vi "MAC-Tester.vi"() -> ()   [LabVIEW 2017]
uses:
  FPGANic/Source.Machine.Settings.ctl
  MAC.Events.ctl
  <vilib>/FPGAPlugInAG/PXIe-6592R/niLvFpga_Open_PXIe-6592R.vi
  <vilib>/rvi/interface/common/dynamic/niFpgaDynamicAddResources.vi
  Globals.vi
  <vilib>/Utility/error.llb/Error Cluster From Error Code.vi
  <vilib>/rvi/errors/niLvFpgaAdjustHostInterfaceError.vi
  <vilib>/FPGAPlugInAG/Dynamic/niLvFpga_Close_Dynamic.vi
  <vilib>/rvi/interface/nirviOpenFPGA/nirviOpenFPGA.xnode
  FPGA Bitfiles/Fpga-Mac-Top.lvbitx
  <vilib>/rvi/interface/nirviMethod/nirviMethod.xnode
  <vilib>/rvi/interface/nirviCloseFPGA/nirviCloseFPGA.xnode
  <vilib>/rvi/errors/niLvFpgaMergeErrorWithErrorCode.vi
  <vilib>/FPGAPlugInAG/Dynamic/niLvFpga_ReadFifo_Dynamic.vi
  <vilib>/FPGAPlugInAG/Dynamic/niLvFpga_WriteFifo_Dynamic.vi
panel:
  in  "MAC & IP":T1={"MAC Address"=[0, 1, 2, 3, 4, 5], "IP Address"=[10, 0, 1, 101]} {"MAC Address" format="%.0x"}
  in  "Ethernet II Params":T2={"Destination MAC"=[0, 2, 201, 85, 8, 68], "Source MAC"=[0, 1, 2, 3, 4, 5], "EtherType"=2048} {"Destination MAC" format="%.0x"; "Source MAC" format="%.02x"; "EtherType" format="%.0x"}
  in  "IPv4 Params":T3={"Destination IP"=[10, 0, 1, 100], "Source IP"=[10, 0, 1, 101], "Protocol"=17}
  in  "UDP Params":T4={"Source Port"=35312, "Destination Port"=35312, "Payload"="ABCD"}
  out "Status":string
  out "error out":errorcluster
  in  "Exit":bool
  in  "Transmit Packet":bool
  in  "Read Packet":bool
  out "RX Data":u8[](array[numeric])=[0, 1, 2, 3, 4, 5, 0, 2, 201, 85, 8, 68, 8, 6, 0, 1, 8, 0, 6, 4, 0, 1, 0, 2, 201, 85, 8, 68, 10, 0, 1, 100, 0, 0, 0, 0, 0, 0, 10, 0, 1, 101, 0, 0, 0, 0, 0, 0, 0, 0, 0, 0, 0, 0, 0, 0, 0, 0, 0, 0, 28, 161, 25, 173] format="%.0x"
  in  "error in":errorcluster
  # "Send Parameters"
  # "Received Data"
  # "NIC Parameters"
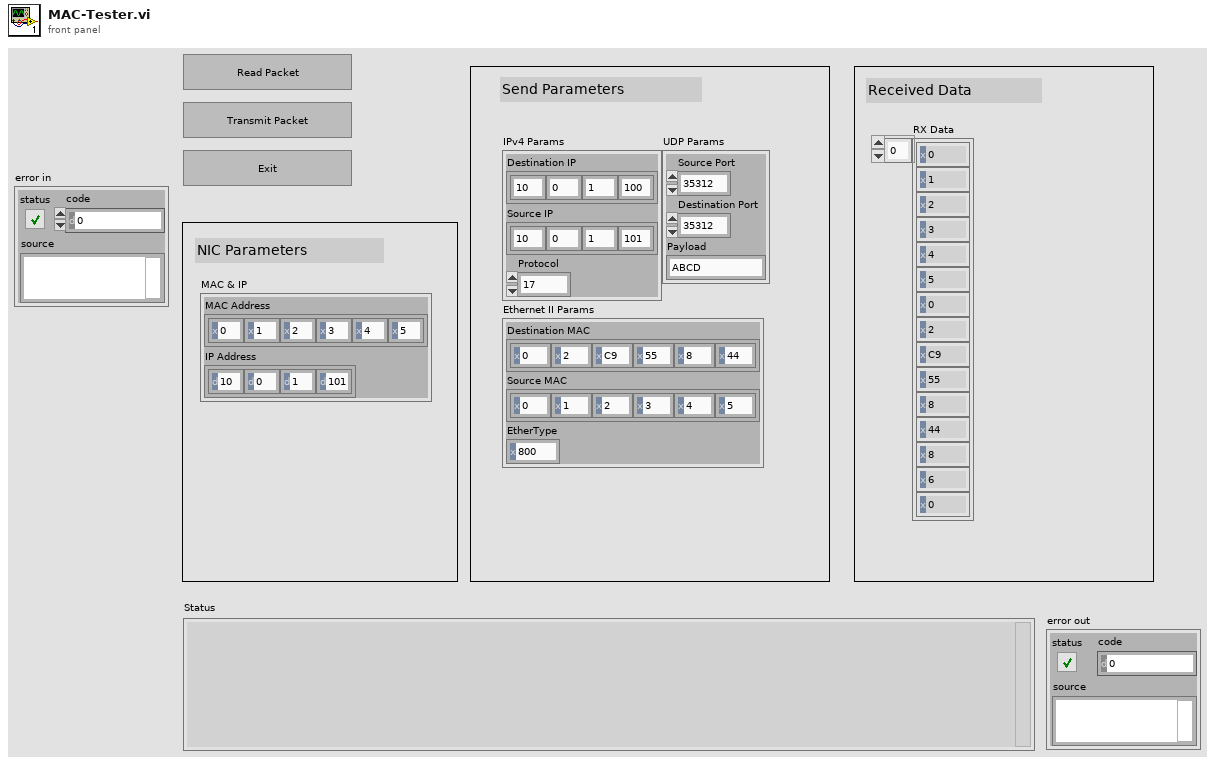
[diagram p1: front panel]
types:
  T1 = typedef "Source.Machine.Settings.ctl" = cluster{"MAC Address":u8[], "IP Address":u8[]}
  T2 = cluster{"Destination MAC":u8[], "Source MAC":u8[], "EtherType":u16}
  T3 = cluster{"Destination IP":u8[], "Source IP":u8[], "Protocol":u8}
  T4 = cluster{"Source Port":u16, "Destination Port":u16, "Payload":string}
  T5 = typedef "MAC.Events.ctl" = enum16{"Open FPGA", "Close FPGA", "Poll RX", "Transmit Packet"}
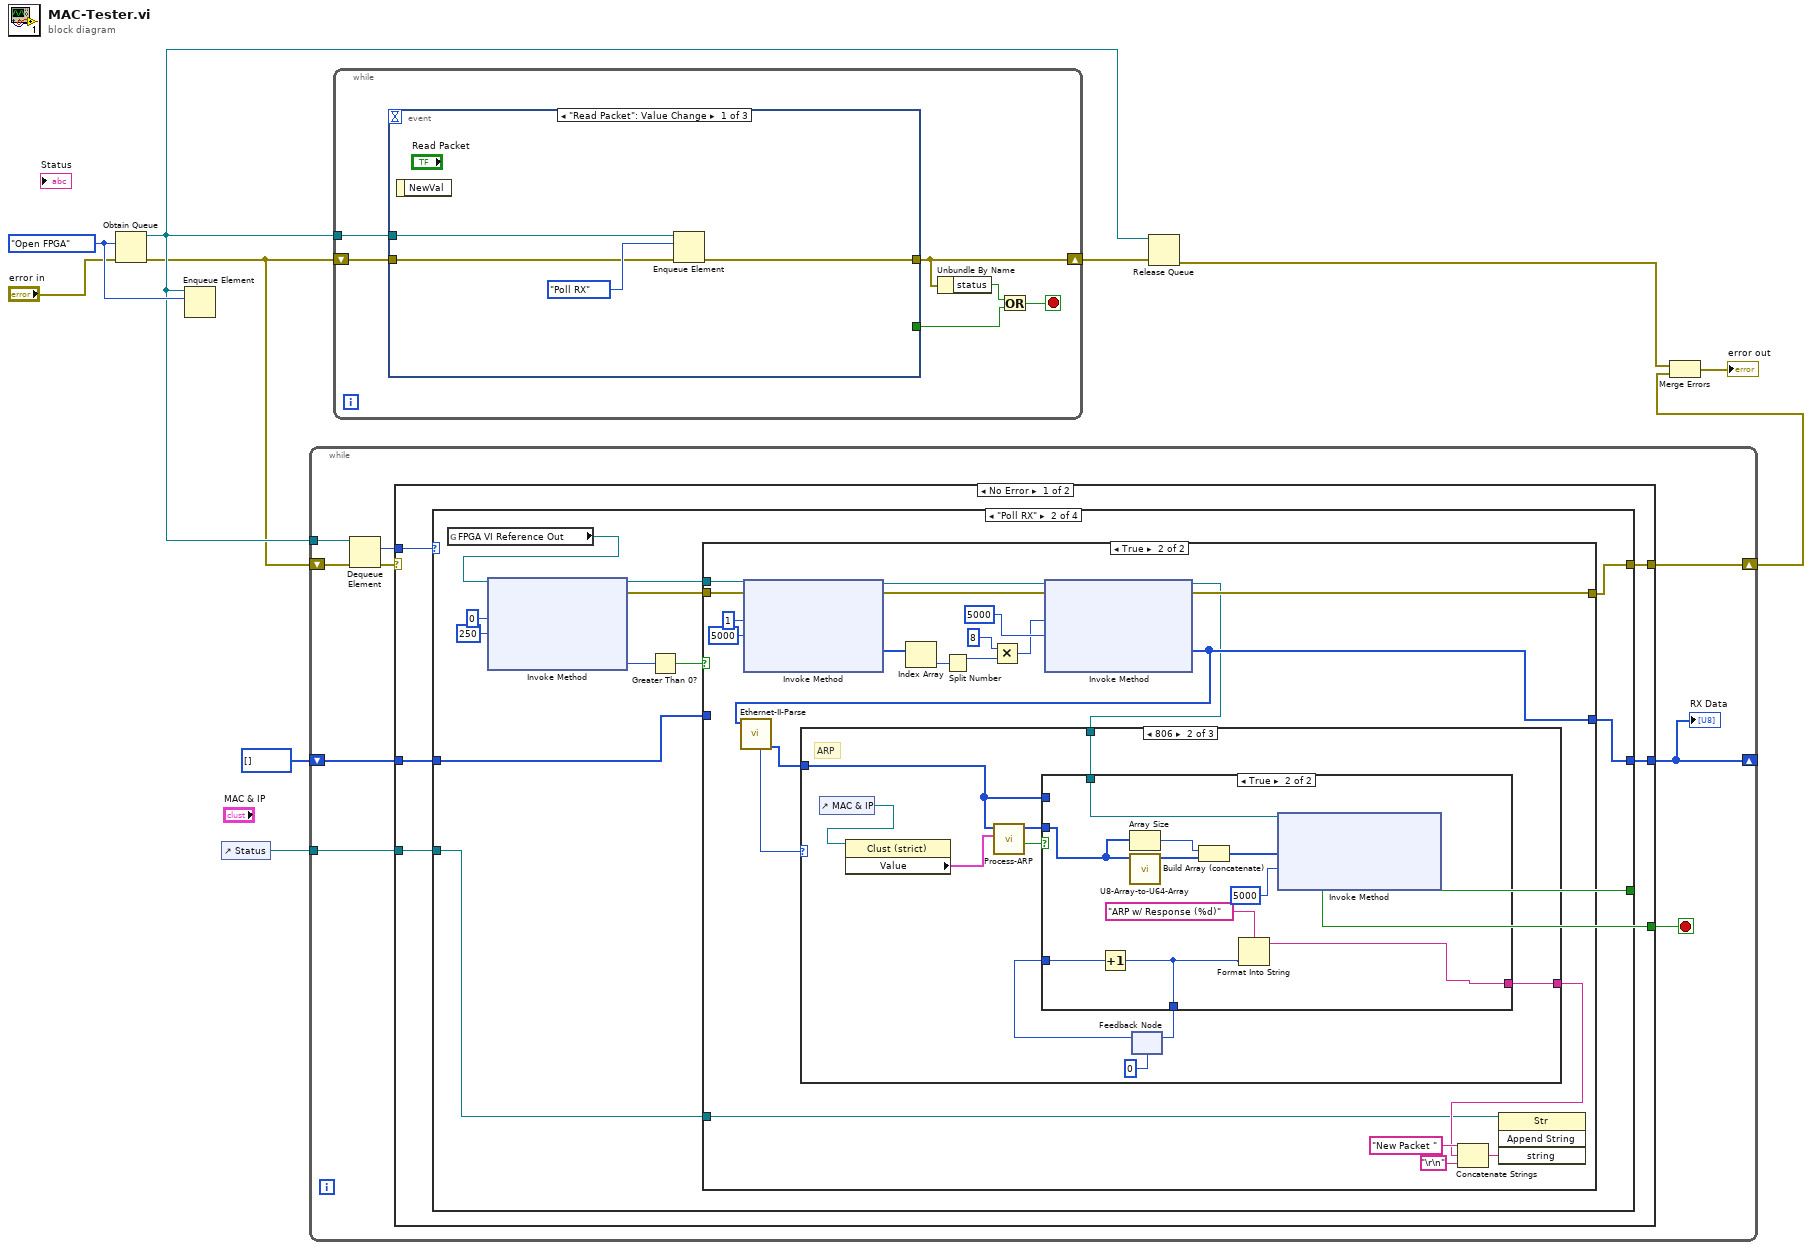
[diagram p0: block diagram]
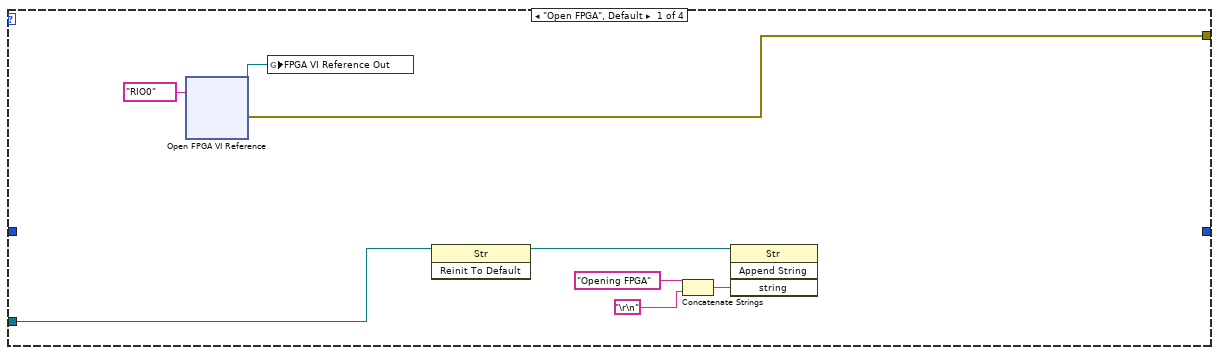
[diagram p2: hidden frame]
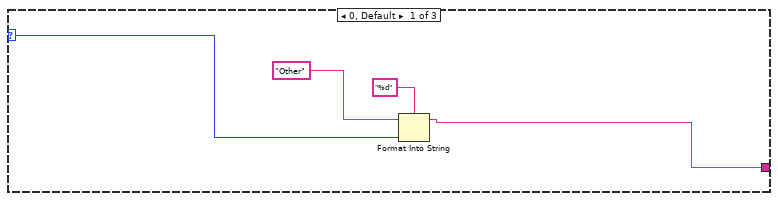
[diagram p4: hidden frame]
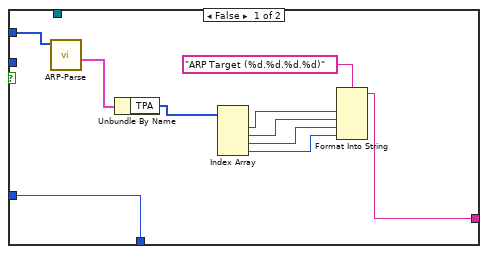
[diagram p5: hidden frame]
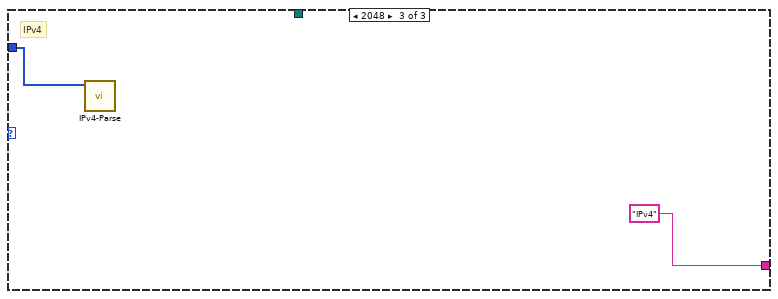
[diagram p6: hidden frame]
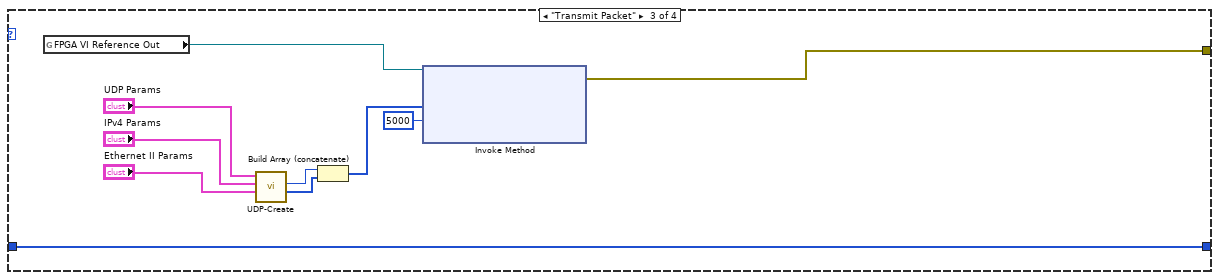
[diagram p7: hidden frame]
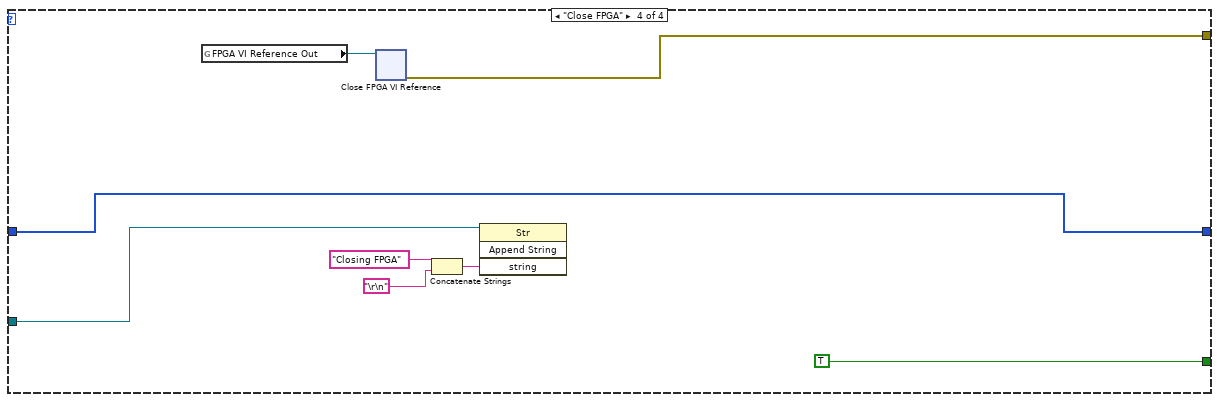
[diagram p8: hidden frame]
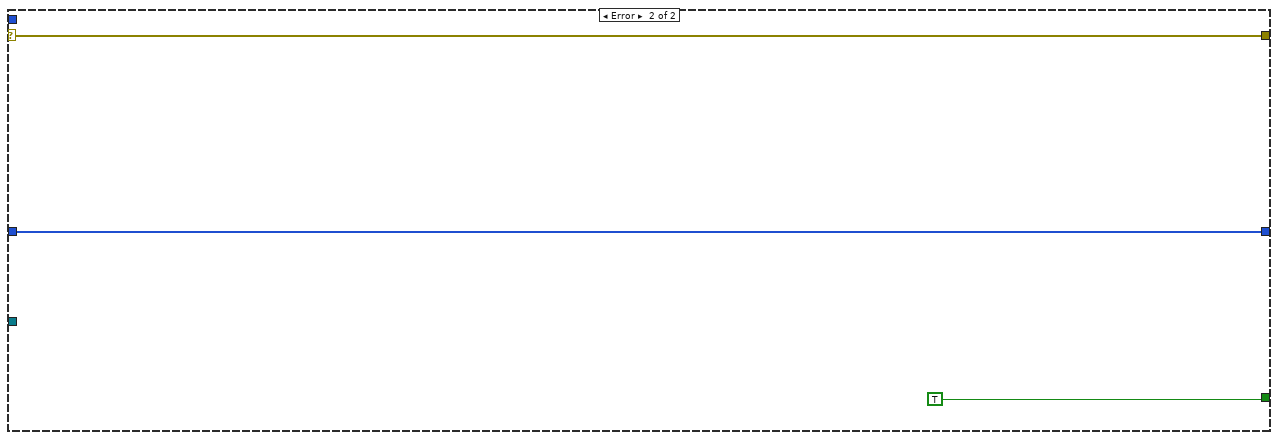
[diagram p9: hidden frame]
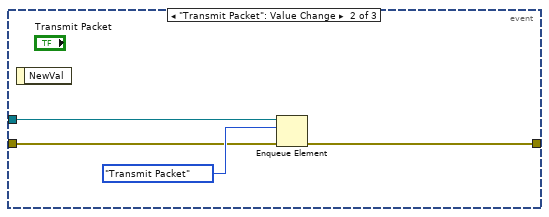
[diagram p10: hidden frame]
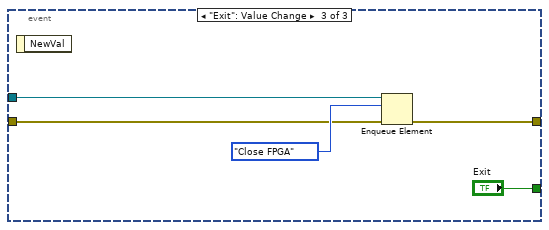
[diagram p11: hidden frame]
diagram:
  w10 = MAC.Events."Open FPGA"
  n1 = Obtain Queue(element data type=w10, error in (no error)="error in") -> (queue out=w8:refnum<queue>, error out=w6:errorcluster)  [unwired: 3 in, 1 out]
  n2 = Enqueue Element(queue=w8, element=w10) -> ()  [unwired: 2 in, 3 out]
  n3 = control-ref of="Status"() -> (w4:refnum<vi>)
  n4 = while {
    tunnel: w8 -> [w19]
    shift-right: [w13] -> w3
    shift-left: w6 -> [w15]
    shift-right: [w12] -> _
    shift-left: u8[] [] -> [w14]
    tunnel: w4 -> [w11]
    stop <- w16 stop-if-true
    n5 = Dequeue Element(queue=w19, error in (no error)=w15) -> (element=w17:T5, error out=w18:errorcluster)  [unwired: 1 in, 2 out]
    n6 = case shown="No Error" w18 {
      selector: w18 -> [_ w123]
      tunnel: w17 -> [w25 _]
      tunnel: [w24 TRUE] -> w16
      tunnel: [w23 w123] -> w13
      tunnel: w14 -> [w22 w124]
      tunnel: [w21 w124] -> w12
      tunnel: w11 -> [w20 _]
      frame No Error {
        n7 = case shown="\"Poll RX\"" w25 {
          tunnel: [_ _ _ TRUE] -> w24
          tunnel: [w33 w36 w106 w121] -> w23
          tunnel: w22 -> [_ w38 w114 w116]
          tunnel: [_ w37 w114 w116] -> w21
          tunnel: w20 -> [w29 w35 _ w117]
          frame "Open FPGA", Default {
            n8 = xnode "Open FPGA VI Reference"("resource name"=tag "RIO0") -> ("FPGA VI Reference Out"=w26:refnum<k20>, "error out"=w33:errorcluster)  [unwired: 1 in]
            n9 = global write "Globals.vi" "FPGA VI Reference Out"(w26) -> ()
            n10 = invoke class="Str" method="Reinit To Default"(reference=w29) -> (reference out=w28:refnum<vi>)  [unwired: 2 in, 2 out]
            n11 = Concatenate Strings("Opening FPGA" ("string"), "\r\n") -> (w32:string)
            n12 = invoke class="Str" method="Append String"(reference=w28, "string"=w32) -> ()  [unwired: 2 in, 4 out]
          }
          frame "Poll RX" {
            n13 = global read "Globals.vi" "FPGA VI Reference Out"() -> (w34:refnum<k20>)
            n14 = xnode "Invoke Method"("FPGA VI Reference In"=w34, "Number of Elements"=u32 0, "Timeout (ms)"=250) -> ("FPGA VI Reference Out"=w40:refnum<k20>, "error out"=w39:errorcluster, "Elements Remaining"=w42:u32)  [unwired: 1 in, 1 out]
            n15 = Greater Than 0?(x=w42) -> (x > 0?=w41:bool)
            n16 = case shown="True" w41 {
              tunnel: w40 -> [_ w66]
              tunnel: w39 -> [w45 w65]
              tunnel: w38 -> [w46 _]
              tunnel: [w46 w50] -> w37
              tunnel: [w45 w59] -> w36
              tunnel: w35 -> [_ w48]
              frame False {
              }
              frame True {
                n17 = xnode "Invoke Method"("FPGA VI Reference In"=w66, "error in"=w65, "Number of Elements"=u32 1, "Timeout (ms)"=5000) -> ("FPGA VI Reference Out"=w62:refnum<k20>, "error out"=w63:errorcluster, "Data"=w64:u32[])  [unwired: 1 out]
                n18 = Index Array(array=w64) -> (element=w61:u32)  [unwired: 1 in]
                n19 = Split Number(x=w61) -> (hi(x)=w55:u16)  [unwired: 1 out]
                n20 = Multiply(x=u16 8 ("y"), y=w55) -> (x*y=w58:u16)
                n21 = xnode "Invoke Method"("FPGA VI Reference In"=w62, "error in"=w63, "Number of Elements"=w58, "Timeout (ms)"=5000) -> ("FPGA VI Reference Out"=w49:refnum<k20>, "error out"=w59:errorcluster, "Data"=w50:u8[])  [unwired: 1 out]
                n22 = call "Ethernet-II-Parse.vi"("Input Frame"=w50) -> ("Payload"=w47:u8[], "EtherType"=w53:u16)  [unwired: 6 in, 3 out]
                n23 = case shown="806" w53 {
                  selector: w53 -> [w72 _ _]
                  tunnel: [w69 w82 "IPv4" ("string")] -> w51
                  tunnel: w47 -> [_ w75 w103]
                  tunnel: w49 -> [_ w79 _]
                  frame 0, Default {
                    n24 = Format Into String(format string="%d", initial string="Other" ("string"), w72) -> (resulting string=w69:string)  [unwired: 1 in, 1 out]
                  }
                  frame 2054 {
                    # "ARP"
                    n25 = control-ref of="MAC & IP"() -> (w73:refnum<vi>)
                    n26 = property class="Clust (strict)"(reference=w73) -> ("Value"=w74:T1)  [unwired: 1 in, 2 out]
                    n27 = call "Process-ARP.vi"("Source Machine\nSettings"=w74, "Frame (in)"=w75) -> ("Response\nNeeded?"=w81:bool, "ARP Response"=w80:u8[])  [unwired: 8 in]
                    n28 = feedback #1(0) -> (w76:i32)
                    n29 = case shown="True" w81 {
                      tunnel: [w89 w93] -> w82
                      tunnel: w80 -> [_ w100]
                      tunnel: w79 -> [_ w101]
                      tunnel: [w92 w95] -> w77
                      tunnel: w76 -> [w92 w96]
                      tunnel: w75 -> [w91 _]
                      frame False {
                        n30 = call "ARP-Parse.vi"("Frame (in)"=w91) -> ("Target"=w88:cluster{"THA":u8[], "TPA":u8[]})  [unwired: 8 in, 2 out]
                        n31 = Unbundle By Name(w88) -> ("TPA"=w87:u8[])
                        n32 = Index Array(array=w87) -> (element #1=w86:u8, element #2=w83:u8, element #3=w84:u8, element #4=w85:u8)  [unwired: 4 in]
                        n33 = Format Into String(format string="ARP Target (%d.%d.%d.%d)", w86, w83, w84, w85) -> (resulting string=w89:string)  [unwired: 2 in, 1 out]
                      }
                      frame True {
                        n34 = Increment(x=w96) -> (x+1=w95:i32)
                        n35 = Array Size(array=w100) -> (size(s)=w98:i32)
                        n36 = call "U8-Array-to-U64-Array.vi"("Frame U8[] in"=w100) -> ("Frame U64[] out"=w99:u64[])  [unwired: 10 in]
                        n37 = Build Array (concatenate)(w98, w99) -> (w97:u64[])
                        n38 = Format Into String(format string="ARP w/ Response (%d)", w95) -> (resulting string=w93:string)  [unwired: 2 in, 1 out]
                        n39 = xnode "Invoke Method"("FPGA VI Reference In"=w101, "Data"=w97, "Timeout (ms)"=5000) -> ()  [unwired: 1 in, 3 out]
                      }
                    }
                    n40 = feedback-in #1(w77) -> ()
                  }
                  frame 2048 {
                    # "IPv4"
                    n41 = call "IPv4-Parse.vi"("IPv4 Packet (in)"=w103) -> ()  [unwired: 8 in, 3 out]
                  }
                }
                n42 = Concatenate Strings("New Packet " ("string"), w51, "\r\n") -> (w57:string)
                n43 = invoke class="Str" method="Append String"(reference=w48, "string"=w57) -> ()  [unwired: 2 in, 4 out]
              }
            }
          }
          frame "Transmit Packet" {
            n44 = global read "Globals.vi" "FPGA VI Reference Out"() -> (w105:refnum<k20>)
            n45 = call "UDP-Create.vi"("Ethernet II Params"="Ethernet II Params", "IPv4 Params"="IPv4 Params", "UDP Params"="UDP Params") -> ("Ethernet Frame\nU64"=w109:u64[], "Ethernet Frame\nsize"=w110:i32)  [unwired: 6 in, 1 out]
            n46 = Build Array (concatenate)(w110, w109) -> (w108:u64[])
            n47 = xnode "Invoke Method"("FPGA VI Reference In"=w105, "Data"=w108, "Timeout (ms)"=5000) -> ("error out"=w106:errorcluster)  [unwired: 1 in, 2 out]
          }
          frame "Close FPGA" {
            n48 = global read "Globals.vi" "FPGA VI Reference Out"() -> (w115:refnum<k20>)
            n49 = xnode "Close FPGA VI Reference"("FPGA VI Reference In"=w115) -> ("error out"=w121:errorcluster)  [unwired: 1 in]
            n50 = Concatenate Strings("Closing FPGA" ("string"), "\r\n") -> (w120:string)
            n51 = invoke class="Str" method="Append String"(reference=w117, "string"=w120) -> ()  [unwired: 2 in, 4 out]
          }
        }
      }
      frame Error {
      }
    }
    "RX Data" <- w12
  }
  n52 = while {
    tunnel: w8 -> [w131]
    shift-right: [w126] -> w9
    shift-left: w6 -> [w127]
    stop <- w129 stop-if-true
    n53 = event shown="[0] \"Read Packet\": Value Change" {
      selector: _ -> [_ _ _]
      dyn-events: _ -> [_ _ _]
      timeout: _ -> [_ _ _]
      tunnel: w131 -> [w135 w138 w143]
      tunnel: [w133 w136 w142] -> w126
      tunnel: [_ _ "Exit"] -> w128
      tunnel: w127 -> [w132 w137 w140]
      event "Read Packet": Value Change {
        n54 = event-data() -> ()  [unwired: 1 in, 1 out]
        n55 = Enqueue Element(queue=w135, element=MAC.Events."Poll RX", error in (no error)=w132) -> (error out=w133:errorcluster)  [unwired: 1 in, 2 out]
      }
      event "Transmit Packet": Value Change {
        n56 = event-data() -> ()  [unwired: 1 in, 1 out]
        n57 = Enqueue Element(queue=w138, element=MAC.Events."Transmit Packet", error in (no error)=w137) -> (error out=w136:errorcluster)  [unwired: 1 in, 2 out]
      }
      event "Exit": Value Change {
        n58 = event-data() -> ()  [unwired: 1 in, 1 out]
        n59 = Enqueue Element(queue=w143, element=MAC.Events."Close FPGA", error in (no error)=w140) -> (error out=w142:errorcluster)  [unwired: 1 in, 2 out]
      }
    }
    n60 = Unbundle By Name(w126) -> ("status"=w130:bool)
    n61 = Or(x=w130, y=w128) -> (x .or. y?=w129:bool)
  }
  n62 = Release Queue(queue=w8, error in (no error)=w9) -> (error out=w1:errorcluster)  [unwired: 1 in, 2 out]
  n63 = Merge Errors(w1, w3) -> (→"error out":errorcluster)
